vi "read_machine_parameters_mt_connect (SubVI).vi"(8 "URL 2":string="http://amrcadp:5000/current/", 10 "error in (no error) 3":errorcluster) -> (0 "error out 3":errorcluster, 3 "Machine Data":T1)   [LabVIEW 2017]
uses:
  <vilib>/addons/internet/NI_InternetTK_Core_VIs.lvlib
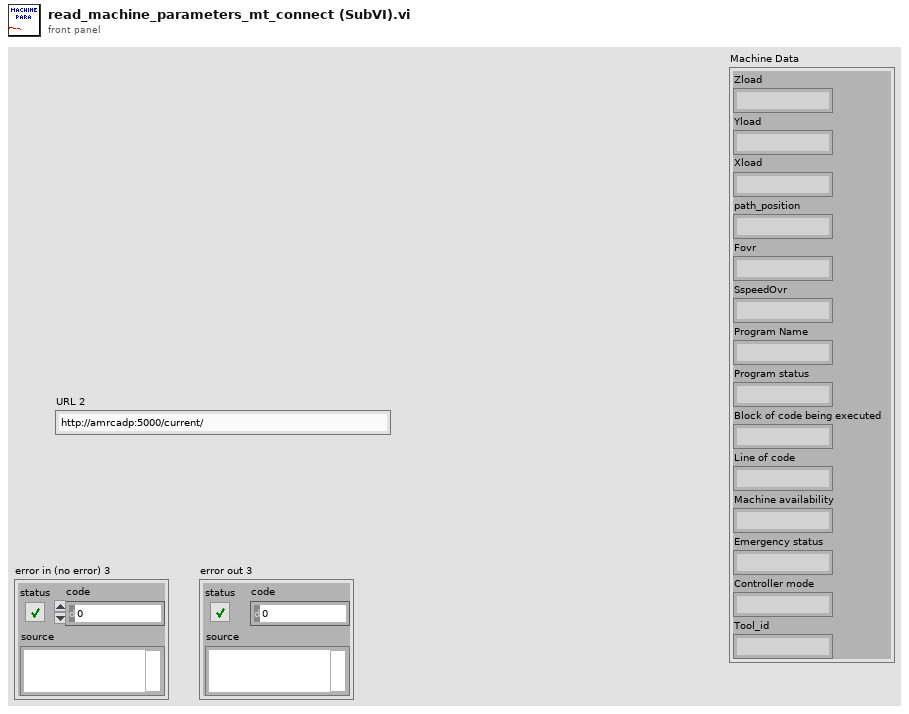
[diagram p1: front panel]
types:
  T1 = cluster{"Zload":string, "Yload":string, "Xload":string, "path_position":string, "Fovr":string, "SspeedOvr":string, "Program Name":string, "Program status":string, "Block of code being executed":string, "Line of code":string, "Machine availability":string, "Emergency status":string, "Controller mode":string, "Tool_id":string}
  T2 = cluster{"Result XML":string, "Result XML":string, "Result XML":string, "Result XML":string, "Result XML":string, "Result XML":string, "Result XML":string, "Result XML":string, "Result XML":string, "Result XML":string, "Result XML":string, "Result XML":string, "Result XML":string, "Result XML":string}
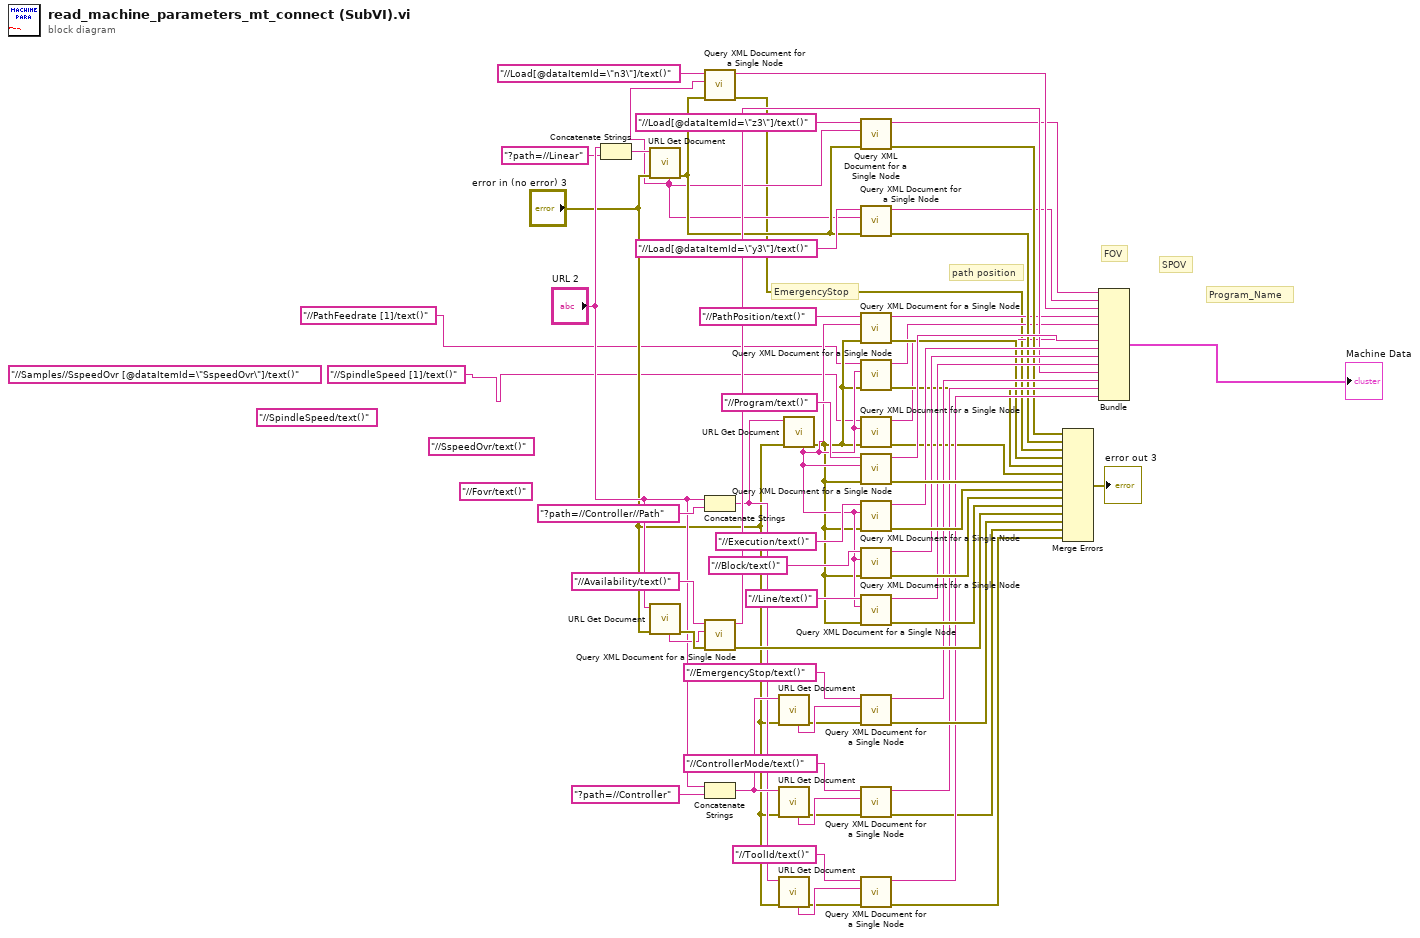
[diagram p0: block diagram]
diagram:
  (unwired) "//SspeedOvr/text()" ("XPath expression")
  (unwired) "//Fovr/text()" ("XPath expression")
  (unwired) "//SpindleSpeed/text()" ("XPath expression")
  (unwired) "//Samples//SspeedOvr [@dataItemId=\"SspeedOvr\"]/text()" ("XPath expression")
  # "Program_Name"
  # "SPOV"
  # "FOV"
  # "path position"
  # "EmergencyStop"
  n1 = Concatenate Strings("URL 2", "?path=//Linear" ("string")) -> (w21:string)
  n2 = call <vilib>:"URL Get Document.vi"("error in (no error)"="error in (no error) 3", "URL"=w21) -> ("error out"=w18:errorcluster, "content"=w6:string)  [unwired: 5 in, 3 out]
  n3 = call <vilib>:"URL Get Document.vi"("error in (no error)"="error in (no error) 3", "URL"="URL 2") -> ("error out"=w60:errorcluster, "content"=w58:string)  [unwired: 5 in, 3 out]
  n4 = call "Query XML Document for a Single Node.vi"("error in (no error)"=w18, "XML document"=w6, "XPath expression"="//Load[@dataItemId=\"n3\"]/text()") -> ("error out"=w3:errorcluster, "Result XML"=w9:string)  [unwired: 6 in, 1 out]
  n5 = Concatenate Strings("URL 2", "?path=//Controller//Path" ("string")) -> (w26:string)
  n6 = call "Query XML Document for a Single Node.vi"("error in (no error)"=w60, "XML document"=w58, "XPath expression"="//Availability/text()") -> ("error out"=w46:errorcluster, "Result XML"=w39:string)  [unwired: 6 in, 1 out]
  n7 = Concatenate Strings("URL 2", "?path=//Controller" ("string")) -> (w51:string)
  n8 = call <vilib>:"URL Get Document.vi"("error in (no error)"="error in (no error) 3", "URL"=w51) -> ("error out"=w33:errorcluster, "content"=w57:string)  [unwired: 5 in, 3 out]
  n9 = call <vilib>:"URL Get Document.vi"("error in (no error)"="error in (no error) 3", "URL"=w51) -> ("error out"=w32:errorcluster, "content"=w55:string)  [unwired: 5 in, 3 out]
  n10 = call <vilib>:"URL Get Document.vi"("error in (no error)"="error in (no error) 3", "URL"=w26) -> ("error out"=w31:errorcluster, "content"=w36:string)  [unwired: 5 in, 3 out]
  n11 = call <vilib>:"URL Get Document.vi"("error in (no error)"="error in (no error) 3", "URL"=w26) -> ("error out"=w15:errorcluster, "content"=w16:string)  [unwired: 5 in, 3 out]
  n12 = call "Query XML Document for a Single Node.vi"("error in (no error)"=w18, "XML document"=w6, "XPath expression"="//Load[@dataItemId=\"z3\"]/text()") -> ("error out"=w12:errorcluster, "Result XML"=w7:string)  [unwired: 6 in, 1 out]
  n13 = call "Query XML Document for a Single Node.vi"("error in (no error)"=w18, "XML document"=w6, "XPath expression"="//Load[@dataItemId=\"y3\"]/text()") -> ("error out"=w13:errorcluster, "Result XML"=w8:string)  [unwired: 6 in, 1 out]
  n14 = call "Query XML Document for a Single Node.vi"("error in (no error)"=w15, "XML document"=w16, "XPath expression"="//PathPosition/text()") -> ("error out"=w14:errorcluster, "Result XML"=w4:string)  [unwired: 6 in, 1 out]
  n15 = call "Query XML Document for a Single Node.vi"("error in (no error)"=w15, "XML document"=w16, "XPath expression"="//PathFeedrate [1]/text()") -> ("error out"=w27:errorcluster, "Result XML"=w10:string)  [unwired: 6 in, 1 out]
  n16 = call "Query XML Document for a Single Node.vi"("error in (no error)"=w15, "XML document"=w16, "XPath expression"="//SpindleSpeed [1]/text()") -> ("error out"=w28:errorcluster, "Result XML"=w11:string)  [unwired: 6 in, 1 out]
  n17 = call "Query XML Document for a Single Node.vi"("error in (no error)"=w15, "XML document"=w16, "XPath expression"="//Program/text()") -> ("error out"=w50:errorcluster, "Result XML"=w43:string)  [unwired: 6 in, 1 out]
  n18 = call "Query XML Document for a Single Node.vi"("error in (no error)"=w15, "XML document"=w16, "XPath expression"="//Execution/text()") -> ("error out"=w49:errorcluster, "Result XML"=w42:string)  [unwired: 6 in, 1 out]
  n19 = call "Query XML Document for a Single Node.vi"("error in (no error)"=w15, "XML document"=w16, "XPath expression"="//Block/text()") -> ("error out"=w48:errorcluster, "Result XML"=w41:string)  [unwired: 6 in, 1 out]
  n20 = call "Query XML Document for a Single Node.vi"("error in (no error)"=w15, "XML document"=w16, "XPath expression"="//Line/text()") -> ("error out"=w47:errorcluster, "Result XML"=w40:string)  [unwired: 6 in, 1 out]
  n21 = call "Query XML Document for a Single Node.vi"("error in (no error)"=w33, "XML document"=w57, "XPath expression"="//EmergencyStop/text()") -> ("error out"=w45:errorcluster, "Result XML"=w38:string)  [unwired: 6 in, 1 out]
  n22 = call "Query XML Document for a Single Node.vi"("error in (no error)"=w32, "XML document"=w55, "XPath expression"="//ControllerMode/text()") -> ("error out"=w30:errorcluster, "Result XML"=w37:string)  [unwired: 6 in, 1 out]
  n23 = call "Query XML Document for a Single Node.vi"("error in (no error)"=w31, "XML document"=w36, "XPath expression"="//ToolId/text()") -> ("error out"=w29:errorcluster, "Result XML"=w34:string)  [unwired: 6 in, 1 out]
  n24 = Merge Errors(w12, w13, w3, w14, w27, w28, w50, w49, w48, w47, w46, w45, w30, w29) -> (→"error out 3":errorcluster)
  n25 = Bundle("Result XML"=w7, "Result XML"=w8, "Result XML"=w9, "Result XML"=w4, "Result XML"=w10, "Result XML"=w11, "Result XML"=w43, "Result XML"=w42, "Result XML"=w41, "Result XML"=w40, "Result XML"=w39, "Result XML"=w38, "Result XML"=w37, "Result XML"=w34) -> (→"Machine Data":T2)  [unwired: 1 in]
